vi "Create Report.vi"(8 "error in (no error)":errorcluster, 11 "Report Generator in":refnum<class "Report Generator.lvclass">) -> (0 "error out":errorcluster, 3 "Report Generator out":refnum<class "Report Generator.lvclass">)   [LabVIEW 2023, in "Report Generator.lvlib" / "Report Generator.lvclass"]
doc: "This parent class method creates the default data directory for the test file and creates a unique file name by calling <b></b>\n\nIt follows this by calling the override method <b>Open Report</b> which descendant classes must override to create the appropriate file/extension.\n\nThe routine checks the error terminal to determine if the report was opened, and asserts/deasserts the <b>IsOpen</b> flag as necessary"
uses:
  Library/Report Generator.lvclass
  Library/Report Generator.lvclass/Report Generator.ctl
  builds/Framework/Engine.lvlibp/Engine/Library/Engine.lvclass
  C:/Users/Public/Documents/Development/builds/Main/Docking.lvlibp/Prime Panel/PrimeDock.lvclass
  C:/Users/Public/Documents/Development/builds/Main/Docking.lvlibp/Docking/Docking.lvclass
  C:/Users/Public/Documents/Development/builds/Framework/Engine.lvlibp/Managed Actor/Library/Managed Actor.lvclass
  C:/Users/Public/Documents/Development/builds/Framework/Engine.lvlibp/Engine/Library/Engine.lvclass
  C:/Users/Public/Documents/Development/builds/Framework/Panel Manager.lvlibp/Library/Panel Actor.lvclass
  C:/Users/Public/Documents/Development/builds/Framework/Monitored Actor.lvlibp/Actor Monitor/Actor Monitor/Actor Monitor.lvclass
  C:/Users/Public/Documents/Development/builds/Framework/Actor Framework.lvlibp/1abvi3w/vi.lib/ActorFramework/Actor/Actor.lvclass
  C:/Users/Public/Documents/Development/Application/Prime Panels/Report Generator/Library/Report Generator.lvclass
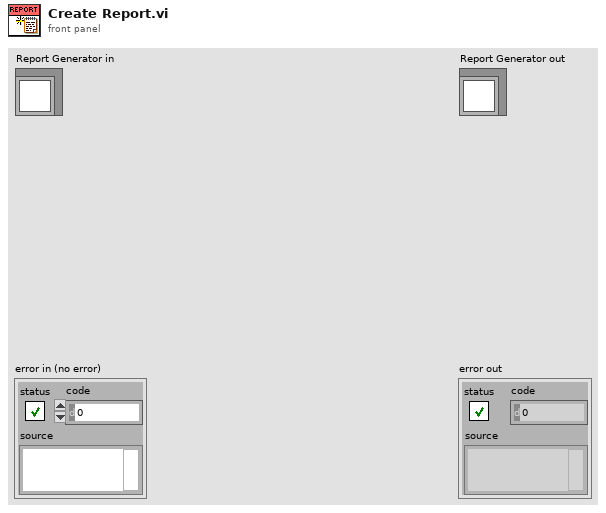
[diagram p1: front panel]
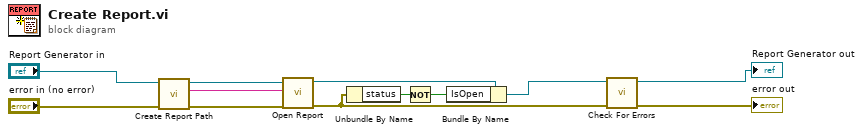
[diagram p0: block diagram]
diagram:
  n1 = call "Create Report Path.vi"("error in (no error)"="error in (no error)", "Report Generator in"="Report Generator in") -> ("error out"=w10:errorcluster, "Unique Test Name"=w8:string, "Report Generator out"=w9:refnum<class "Report Generator.lvclass">)  [unwired: 7 in]
  n2 = call-dynamic "Open Report.vi"("error in (no error)"=w10, "UniqueFileName(NoExt)"=w8, "Report Generator in"=w9) -> ("error out"=w4:errorcluster, "Report Generator out"=w6:refnum<class "Report Generator.lvclass">)  [unwired: 7 in]
  n3 = Unbundle By Name(w4) -> ("status"=w2:bool)
  n4 = Not(x=w2) -> (.not. x?=w1:bool)
  n5 = Bundle By Name(cluster=w6, "IsOpen"=w1) -> (w3:refnum<class "Report Generator.lvclass">)
  n6 = call "Check For Errors.vi"("error in"=w4, "Engine in"=w3) -> ("error out"=→"error out":errorcluster, "Engine out"=→"Report Generator out":refnum<class "Report Generator.lvclass">)  [unwired: 8 in]
